vi "DecodeMessageFormat.vi"(5 "Messages":u8[](array[numeric])) -> (0 "# of terminals":u8, 2 "CRef Types":T2[](array[typedef]), 3 "Terminal Bounds[]":T1[](array[typedef]))   [LabVIEW 2012]
uses:
  CRef/Core/Master Types.ctl
  <vilib>/Utility/miscctls.llb/LVRectTypeDef.ctl
  CRef/CRef.lvlib
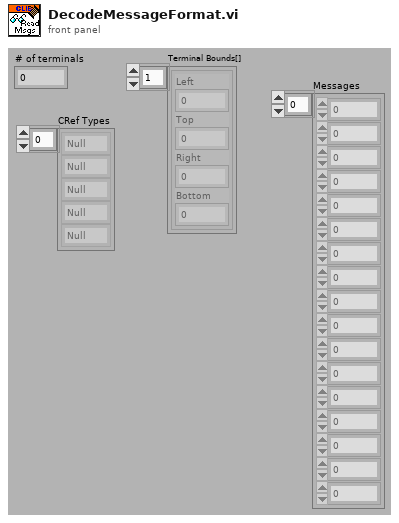
[diagram p1: front panel]
types:
  T1 = typedef "LVRectTypeDef.ctl" = cluster{"Left":i16, "Top":i16, "Right":i16, "Bottom":i16}
  T2 = typedef "CRef.lvlib/Master Types.ctl" = enum8{"Null", "Boolean", "U8", "I8", "U16", "I16", "U32", "I32", "U64", "I64", "Single", "Double", "Extended", "CSG", "CDB", "CXT", "Boolean(Def)", "U8(Def)", "I8(Def)", "U16(Def)", "I16(Def)", "U32(Def)", "I32(Def)", "Reserved Def", "Reserved Def1", "Single(Def)", "Double(Def)", "Reserved Def2", "Reserved Def3", "Reserved Def4", "Reserved Def5", "Unsigned(Def)", "Signed(Def)", "Real(Def)", "Reserved Def6", "Numeric(Def)", "String"}
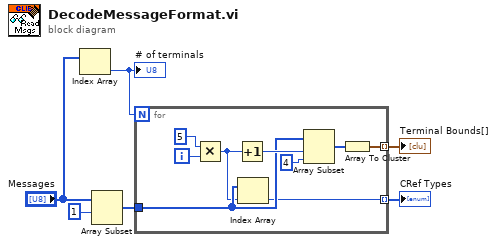
[diagram p0: block diagram]
diagram:
  n1 = Index Array(array="Messages") -> (element=w1:u8)  [unwired: 1 in]
  "# of terminals" <- w1
  n2 = Array Subset(array="Messages", index=1) -> (w4:u8[])  [unwired: 1 in]
  n3 = for {
    N: w1 -> [_]
    tunnel: w4 -> [w9]
    tunnel: [w12] -> w3 mode=indexing
    tunnel: [w7] -> w2 mode=indexing
    i -> [w15]
    n4 = Multiply(x=5, y=w15) -> (x*y=w8:i32)
    n5 = Increment(x=w8) -> (x+1=w11:i32)
    n6 = Index Array(array=w9, index=w8) -> (element=w7:u8)
    n7 = Array Subset(array=w9, index=w11, length=4) -> (w13:u8[])
    n8 = Array To Cluster(array=w13) -> (cluster=w12:cluster{"[0]":u8, "[1]":u8, "[2]":u8, "[3]":u8})
  }
  "CRef Types" <- w2
  "Terminal Bounds[]" <- w3
